vi "Prepare Config Files.vi"(8 "error in":errorcluster, 11 "Project Root":path) -> (0 "error out":errorcluster, 3 "Config":path)   [LabVIEW 2011]
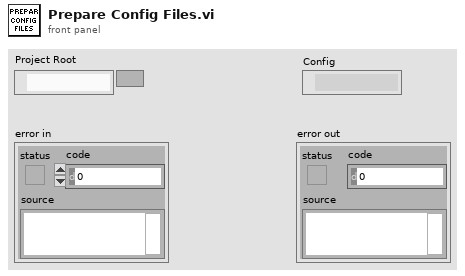
[diagram p1: front panel]
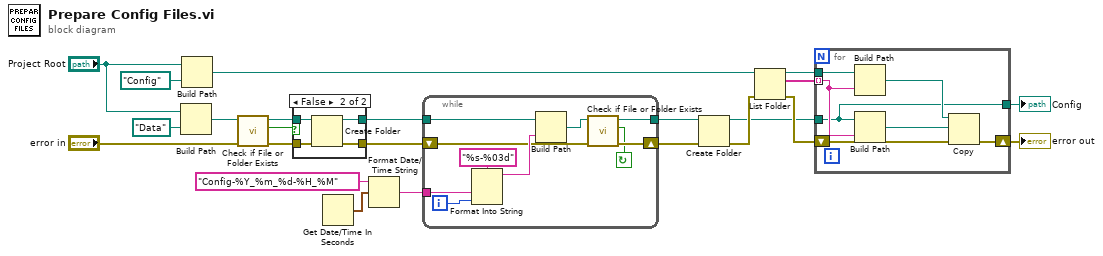
[diagram p0: block diagram]
diagram:
  n1 = Build Path(base path="Project Root", name or relative path=path "Data") -> (appended path=w20:path)
  n2 = Build Path(base path="Project Root", name or relative path=path "Config") -> (appended path=w1:path)
  n3 = call <vilib>:"Check if File or Folder Exists.vi"("error in (no error)"="error in", "path"=w20) -> ("error out"=w18:errorcluster, "file or folder exists?"=w16:bool, "dup path"=w17:path)  [unwired: 7 in]
  n4 = case shown="False" w16 {
    tunnel: [w25 w29] -> w14
    tunnel: [w24 w28] -> w15
    tunnel: w18 -> [w24 w27]
    tunnel: w17 -> [w25 w26]
    frame True {
    }
    frame False {
      n5 = Create Folder(path (use dialog)=w26, error in=w27) -> (created path=w29:path, error out=w28:errorcluster)  [unwired: 1 in, 1 out]
    }
  }
  n6 = Get Date/Time In Seconds() -> (seconds since 1Jan1904=w22:timestamp)
  n7 = Format Date/Time String(time format string (%c)="Config-%Y_%m_%d-%H_%M", seconds (now)=w22) -> (date/time string=w13:string)  [unwired: 1 in]
  n8 = while {
    tunnel: w14 -> [w36]
    tunnel: w13 -> [w37]
    shift-right: [w32] -> w12
    shift-left: w15 -> [w33]
    tunnel: [w30] -> w11
    i -> [w38]
    stop <- w31 continue-if-true
    n9 = Format Into String(format string="%s-%03d", w37, w38) -> (resulting string=w35:string)  [unwired: 2 in, 1 out]
    n10 = Build Path(base path=w36, name or relative path=w35) -> (appended path=w34:path)
    n11 = call <vilib>:"Check if File or Folder Exists.vi"("error in (no error)"=w33, "path"=w34) -> ("error out"=w32:errorcluster, "file or folder exists?"=w31:bool, "dup path"=w30:path)  [unwired: 7 in]
  }
  n12 = Create Folder(path (use dialog)=w11, error in=w12) -> (created path=w6:path, error out=w10:errorcluster)  [unwired: 1 in, 1 out]
  n13 = List Folder(path=w1, error in=w10) -> (path out=w8:path, filenames=w9:string[], error out=w7:errorcluster)  [unwired: 2 in, 1 out]
  n14 = for {
    tunnel: w9 -> [w45] mode=indexing
    tunnel: w8 -> [w46]
    tunnel: w6 -> [w40]
    shift-right: [w41] -> w4
    shift-left: w7 -> [w44]
    tunnel: [w40] -> w5
    n15 = Build Path(base path=w46, name or relative path=w45) -> (appended path=w43:path)
    n16 = Build Path(base path=w40, name or relative path=w45) -> (appended path=w42:path)
    n17 = Copy(8:w44, 10:w42, 11:w43) -> (0:w41:errorcluster)  [unwired: 2 in, 2 out]
  }
  "Config" <- w5
  "error out" <- w4
